vi "Programming Mode.vi"(8 "error in (no error)":errorcluster, 11 "serverName In":string="10.0.18.244") -> (0 "error out":errorcluster, 3 "serverName Out":string="10.0.18.244")   [LabVIEW 2019, in "SEECD System Explorer.lvlib"]
doc: "This VI detects whether or not target local chassis supports \"Slot Programming Mode\" property.\nIf the case, populated slots have current value for the property displayed and user can change property.\nIf not the case, front-panel is not opened."
uses:
  SEECD System Explorer.lvlib
  Type Defs/Slot - Configuration.ctl
  <vilib>/nisyscfg/Close (Resources).vi
  <vilib>/nisyscfg/Close (Filter).vi
  <vilib>/nisyscfg/Close (System).vi
  <vilib>/nisyscfg/nisyscfg.lvlib
panel:
  in  "Slot 7":T1={"Slot"="", "Module Name"="", "Slot Programming Mode"=enum."Don't Modify"} caption="Slot"
  in  "Slot 6":T1={"Slot"="", "Module Name"="", "Slot Programming Mode"=enum."Don't Modify"} caption="Slot"
  in  "Slot 5":T1={"Slot"="", "Module Name"="", "Slot Programming Mode"=enum."Don't Modify"} caption="Slot"
  in  "Slot 4":T1={"Slot"="", "Module Name"="", "Slot Programming Mode"=enum."Don't Modify"} caption="Slot"
  in  "Slot 3":T1={"Slot"="", "Module Name"="", "Slot Programming Mode"=enum."Don't Modify"} caption="Slot"
  in  "Slot 2":T1={"Slot"="", "Module Name"="", "Slot Programming Mode"=enum."Don't Modify"} caption="Slot"
  in  "Slot 1":T1={"Slot"="", "Module Name"="", "Slot Programming Mode"=enum."Don't Modify"} caption="Slot"
  in  "Slot 0":T1={"Slot"="", "Module Name"="", "Slot Programming Mode"=enum."Don't Modify"} caption="Slot"
  in  "User Name":string
  in  "Password":string
  in  "Set all modules to \"Scan Engine\" mode":bool
  in  "Cancel":bool
  in  "OK":bool
  # "Select a programming mode for detected \nmodules and click \"OK\" button."
  # "Module Name"
  # "Programming Mode"
  # "Modules Name"
  # "Slot"
  # "Programming Mode"
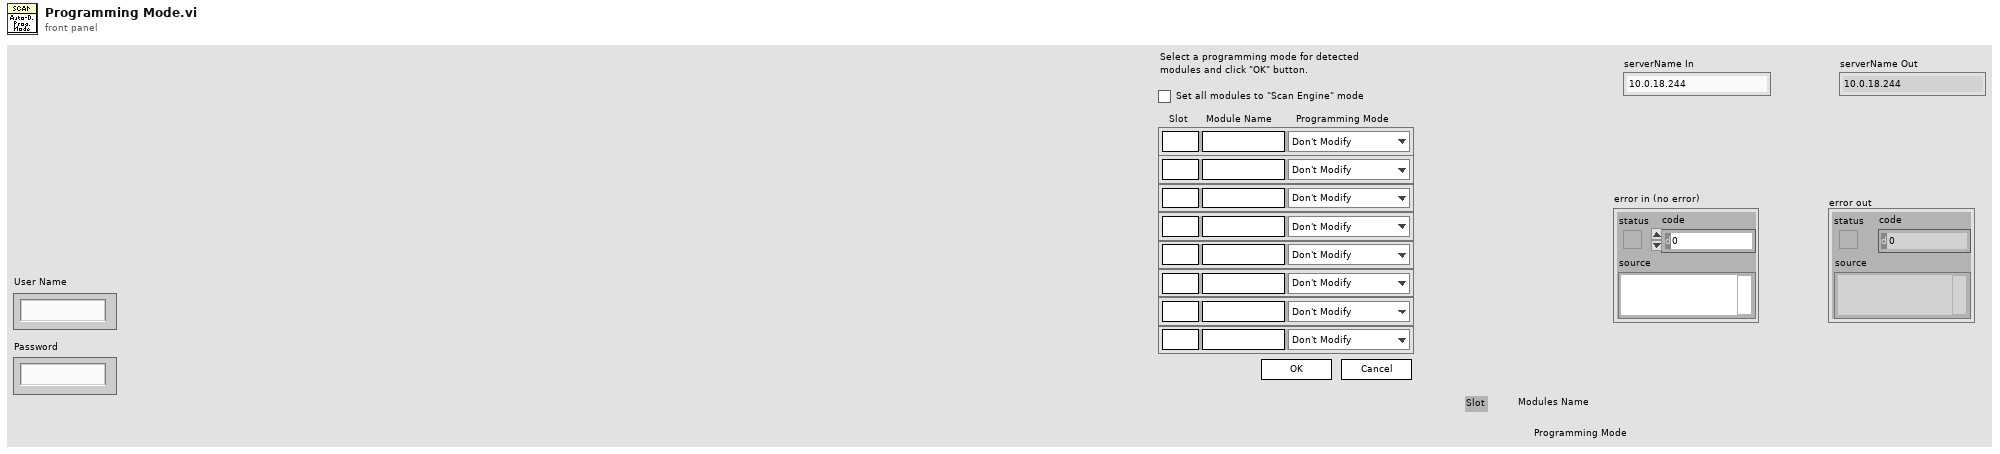
[diagram p1: front panel]
types:
  T1 = typedef "SEECD System Explorer.lvlib/Slot - Configuration.ctl" = cluster{"Slot":string, "Module Name":string, "Slot Programming Mode":enum16{"Scan Engine", "LabVIEW FPGA", "NI-DAQmx", "Don't Modify"}}
  T2 = enum32{"Invalid", "Standard", "Closed", "Hidden", "Minimized", "Maximized"}
  T3 = typedef "SEECD System Explorer.lvlib/Slot Programming Mode.ctl" = enum16{"Scan Engine", "LabVIEW FPGA", "NI-DAQmx", "Don't Modify"}
  T4 = enum16{"Scan Engine", "LabVIEW FPGA", "NI-DAQmx", "Don't Modify"}
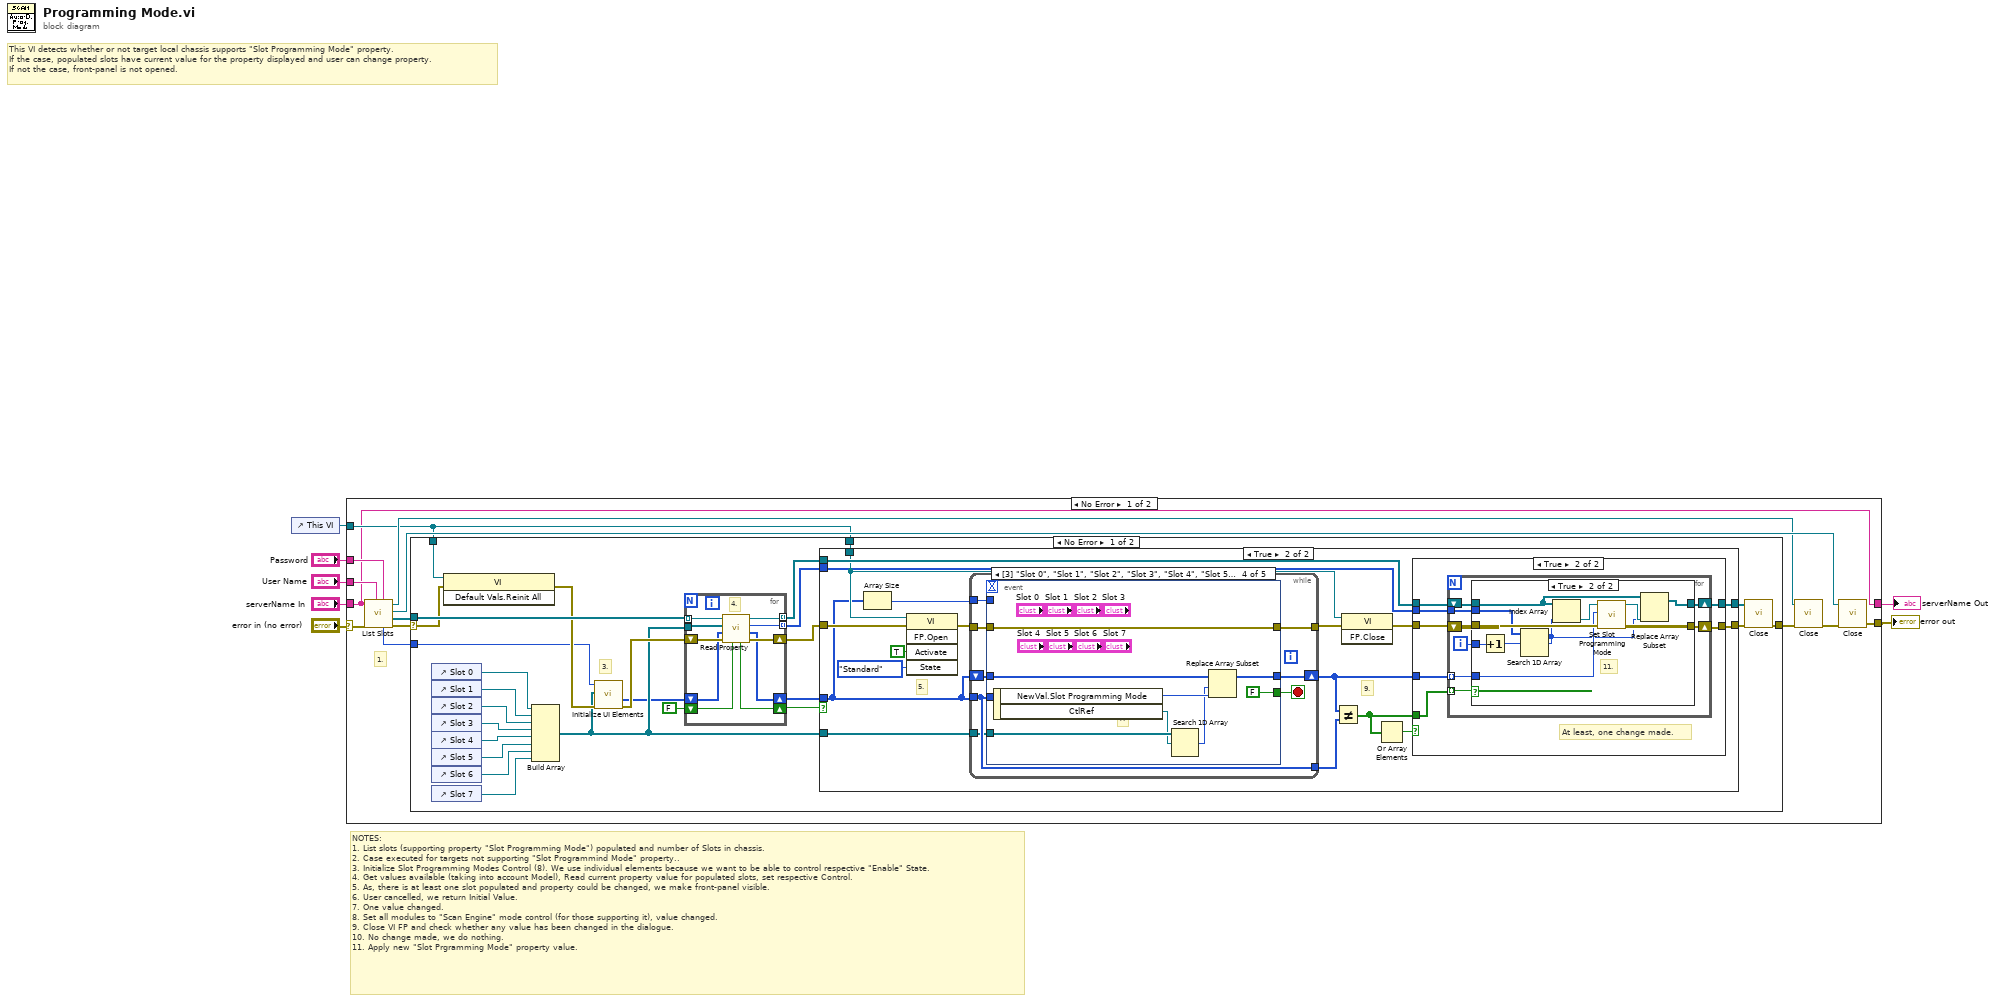
[diagram p0: block diagram]
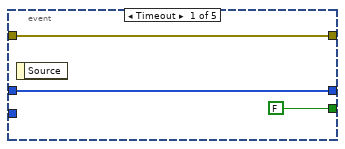
[diagram p3: hidden frame]
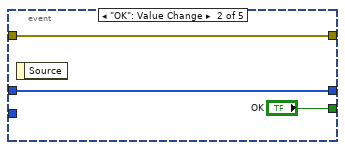
[diagram p4: hidden frame]
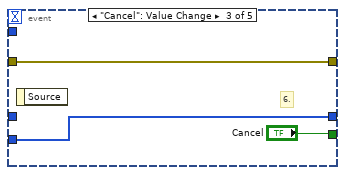
[diagram p5: hidden frame]
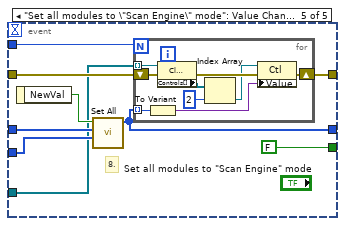
[diagram p6: hidden frame]
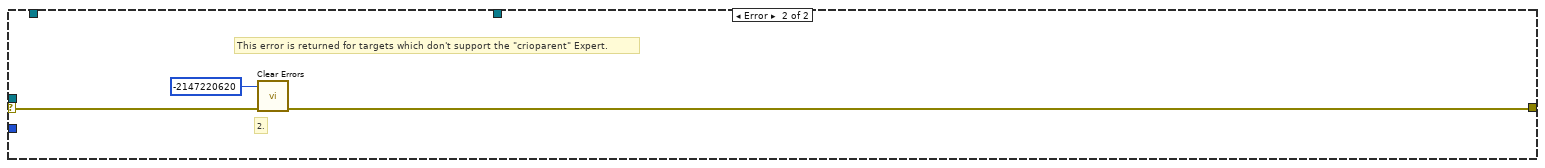
[diagram p9: hidden frame]
diagram:
  # "NOTES:\n1. List slots (supporting property \"Slot Programming Mode\") populated and number of Slots in chassis.\n2. Case executed for targets not supporting \"Slot Programmind Mode\" property..\n3. Initialize Slot Programming Modes Control (8). We use individual elements because we want to be able to control respective \"Enable\" State.\n4. Get values available (taking into account Model), Read current property value for populated slots, set respective Control.\n5. As, there is at least one slot populated and property could be changed, we make front-panel visible.\n6. User cancelled, we return Initial Value.\n7. One value changed.\n8. Set all modules to \"Scan Engine\" mode control (for those supporting it), value changed.\n9. Close VI FP and check whether any value has been changed in the dialogue.\n10. No change made, we do nothing.\n11. Apply new \"Slot Prgramming Mode\" property value."
  # "This VI detects whether or not target local chassis supports \"Slot Programming Mode\" property.\nIf the case, populated slots have current value for the property displayed and user can change property.\nIf not the case, front-panel is not opened."
  n1 = control-ref of="This VI"() -> (w2:refnum<vi>)
  n2 = case shown="No Error" "error in (no error)" {
    selector: "error in (no error)" -> [w19 w154]
    tunnel: "serverName In" -> [w9 w153]
    tunnel: "User Name" -> [w11 _]
    tunnel: "Password" -> [w10 _]
    tunnel: [w20 w154] -> w3
    tunnel: w2 -> [w12 _]
    tunnel: [w9 w153] -> w1
    frame No Error {
      # "1."
      n3 = call "List Slots.vi"("Password"=w10, "User Name"=w11, "error in (no error)"=w19, "serverName In"=w9) -> ("error out"=w14:errorcluster, "Resources out"=w18:refnum<k20>[], "Session out"=w17:refnum<k21>, "Refnum out"=w13:refnum<k20>, "NumSlots"=w8:i32)  [unwired: 3 in]
      n4 = case shown="No Error" w14 {
        selector: w14 -> [w36 w152]
        tunnel: w18 -> [w46 _]
        tunnel: [w42 w150] -> w15
        tunnel: w12 -> [w41 _]
        tunnel: w12 -> [w37 _]
        tunnel: w8 -> [w23 _]
        frame No Error {
          # "3."
          n5 = control-ref of="Slot 0"() -> (w28:refnum<vi>)
          n6 = control-ref of="Slot 1"() -> (w29:refnum<vi>)
          n7 = control-ref of="Slot 2"() -> (w30:refnum<vi>)
          n8 = control-ref of="Slot 3"() -> (w31:refnum<vi>)
          n9 = control-ref of="Slot 4"() -> (w32:refnum<vi>)
          n10 = control-ref of="Slot 5"() -> (w33:refnum<vi>)
          n11 = control-ref of="Slot 6"() -> (w34:refnum<vi>)
          n12 = control-ref of="Slot 7"() -> (w35:refnum<vi>)
          n13 = invoke class="VI" method="Default Vals.Reinit All"(reference=w37, error in=w36) -> (error out=w27:errorcluster)  [unwired: 1 in, 2 out]
          n14 = Build Array(w28, w29, w30, w31, w32, w33, w34, w35) -> (w22:refnum<vi>[])
          n15 = call "Initialize UI Elements.vi"("error in"=w27, "References"=w22, "NumSlots"=w23) -> ("error out"=w26:errorcluster, "Programming Mode Out"=w21:T3[])  [unwired: 7 in]
          n16 = for {
            tunnel: w46 -> [w145] mode=indexing
            shift-right: [w149] -> w43
            shift-left: w26 -> [w148]
            tunnel: [w144] -> w40 mode=indexing
            shift-right: [w141] -> w44
            shift-left: FALSE -> [w147]
            tunnel: w22 -> [w140]
            shift-right: [w142] -> w25
            shift-left: w21 -> [w146]
            tunnel: [w143] -> w24 mode=indexing
            # "4."
            n17 = call "Read Property.vi"("Initialized in"=w147, "error in (no error)"=w148, "Programming Mode In"=w146, "References"=w140, "Refnum in"=w145) -> ("error out"=w149:errorcluster, "Programming Mode Out"=w142:T3[], "Slot"=w143:i32, "Refnum out"=w144:refnum<k20>, "Initialized Out"=w141:bool)  [unwired: 2 in]
          }
          n18 = case shown="True" w44 {
            tunnel: w43 -> [w48 w53]
            tunnel: [w48 w56] -> w38
            tunnel: w25 -> [_ w51]
            tunnel: w41 -> [_ w54]
            tunnel: w40 -> [w47 w61]
            tunnel: [w47 w55] -> w39
            tunnel: w22 -> [_ w52]
            tunnel: w24 -> [_ w49]
            frame False {
            }
            frame True {
              # "9."
              # "5."
              n19 = Array Size(array=w51) -> (size(s)=w50:i32)
              n20 = invoke class="VI" method="FP.Open"(reference=w54, error in=w53, "Activate"=TRUE ("Activate?"), "State"=T2."Standard") -> (error out=w63:errorcluster)  [unwired: 1 in, 4 out]
              n21 = while {
                tunnel: w63 -> [w74]
                tunnel: w51 -> [w71]
                tunnel: [w71] -> w66
                tunnel: [w70] -> w62
                shift-right: [w72] -> w57
                shift-left: w51 -> [w69]
                tunnel: w52 -> [w68]
                tunnel: w50 -> [w67]
                stop <- w73 stop-if-true
                n22 = event shown="[3] \"Slot 0\", \"Slot 1\", \"Slot 2\", \"Slot 3\", \"Slot 4\", \"Slot 5\", \"Slot 6\", \"Slot 7\": Value Change" {
                  selector: _ -> [_ _ _ _ _]
                  dyn-events: _ -> [_ _ _ _ _]
                  timeout: _ -> [_ _ _ _ _]
                  tunnel: w74 -> [w77 w79 w81 w90 w96]
                  tunnel: [FALSE ("Cancel") "OK" "Cancel" FALSE ("Cancel") FALSE ("Cancel")] -> w73
                  tunnel: [w76 w78 w82 w87 w94] -> w72
                  tunnel: w71 -> [_ _ w82 _ w95]
                  tunnel: [w77 w79 w81 w90 w97] -> w70
                  tunnel: w69 -> [w76 w78 _ w89 w98]
                  tunnel: w68 -> [_ _ _ w86 w93]
                  tunnel: w67 -> [_ _ _ _ w92]
                  event Timeout {
                    n23 = event-data() -> ()  [unwired: 1 in, 1 out]
                  }
                  event "OK": Value Change {
                    n24 = event-data() -> ()  [unwired: 1 in, 1 out]
                  }
                  event "Cancel": Value Change {
                    # "6."
                    n25 = event-data() -> ()  [unwired: 1 in, 1 out]
                  }
                  event Value Change {
                    # "7."
                    n26 = event-data() -> ("NewVal.Slot Programming Mode"=w88:T4, "CtlRef"=w84:refnum<vi>)  [unwired: 1 in]
                    n27 = Search 1D Array(1D array=w86, element=w84) -> (index of element=w85:i32)  [unwired: 1 in]
                    n28 = Replace Array Subset(array=w89, new element=w88, index=w85) -> (w87:T3[])
                  }
                  event "Set all modules to \"Scan Engine\" mode": Value Change {
                    # "8."
                    n29 = event-data() -> ("NewVal"=w99:bool)  [unwired: 1 in]
                    n30 = call "Set All.vi"("Init Value"=w95, "Previous Value"=w98, "Set ALL NewVal"=w99) -> ("Value Out"=w94:T3[])  [unwired: 8 in]
                    n31 = for {
                      N: w92 -> [_]
                      tunnel: w94 -> [w102] mode=indexing
                      shift-right: [w103] -> w97
                      shift-left: w96 -> [w109]
                      tunnel: w93 -> [w108] mode=indexing
                      n32 = To Variant(anything=w102) -> (Variant=w101:variant)
                      n33 = property class="Clust (strict)"(reference=w108, error in=w109) -> (error out=w105:errorcluster, "Controls[]"=w107:refnum<vi>[])  [unwired: 1 out]
                      n34 = Index Array(array=w107, index=2) -> (element=w104:refnum<vi>)
                      n35 = property class="Ctl"(reference=w104, error in=w105, "Value"=w101) -> (error out=w103:errorcluster)  [unwired: 1 out]
                    }
                  }
                }
              }
              n36 = Not Equal?(x=w57, y=w66) -> (x != y?=w58:bool[])
              n37 = invoke class="VI" method="FP.Close"(reference=w54, error in=w62) -> (error out=w60:errorcluster)  [unwired: 1 in, 2 out]
              n38 = Or Array Elements(Boolean array=w58) -> (logical OR=w59:bool)
              n39 = case shown="True" w59 {
                tunnel: w61 -> [w110 w118]
                tunnel: w60 -> [w111 w117]
                tunnel: w58 -> [_ w116]
                tunnel: w57 -> [_ w115]
                tunnel: [w111 w114] -> w56
                tunnel: [w110 w113] -> w55
                tunnel: w49 -> [_ w112]
                frame False {
                  # "10."
                  # "Not a single change."
                }
                frame True {
                  # "At least, one change made."
                  n40 = for {
                    tunnel: w116 -> [w126] mode=indexing
                    tunnel: w115 -> [w125] mode=indexing
                    shift-right: [w122] -> w114
                    shift-left: w117 -> [w124]
                    tunnel: w112 -> [w119]
                    shift-right: [w121] -> w113
                    shift-left: w118 -> [w123]
                    i -> [w120]
                    n41 = case shown="True" w126 {
                      tunnel: w125 -> [_ w137]
                      tunnel: w124 -> [w128 w139]
                      tunnel: w123 -> [w127 w131]
                      tunnel: [w128 w138] -> w122
                      tunnel: [w127 w129] -> w121
                      tunnel: w120 -> [_ w135]
                      tunnel: w119 -> [_ w136]
                      frame False {
                      }
                      frame True {
                        # "11."
                        n42 = Increment(x=w135) -> (x+1=w134:i32)
                        n43 = Search 1D Array(1D array=w136, element=w134) -> (index of element=w130:i32)  [unwired: 1 in]
                        n44 = Index Array(array=w131, index=w130) -> (element=w133:refnum<k20>)
                        n45 = call "Set Slot Programming Mode.vi"("error in (no error)"=w139, "Slot Programming Mode"=w137, "Refnum in"=w133) -> ("error out"=w138:errorcluster, "Refnum out"=w132:refnum<k20>)  [unwired: 7 in]
                        n46 = Replace Array Subset(array=w131, new element=w132, index=w130) -> (w129:refnum<k20>[])
                      }
                    }
                  }
                }
              }
            }
          }
          n47 = call-poly <vilib>:"Close.vi"("error in (no error)"=w38, "Resources in"=w39) -> ("error out"=w42:errorcluster)  [unwired: 9 in]
        }
        frame Error {
          # "2."
          # "This error is returned for targets which don't support the \"crioparent\" Expert."
          n48 = call <vilib>:"Clear Errors.vi"("error in (no error)"=w152, "specific error code to clear (0: all)"=-2147220620) -> ("error out"=w150:errorcluster)  [unwired: 4 in, 1 out]
        }
      }
      n49 = call-poly <vilib>:"Close.vi"("error in (no error)"=w15, "Filter in"=w13) -> ("error out"=w16:errorcluster)  [unwired: 9 in]
      n50 = call-poly <vilib>:"Close.vi"("error in (no error)"=w16, "Session in"=w17) -> ("error out"=w20:errorcluster)  [unwired: 9 in]
    }
    frame Error {
    }
  }
  "error out" <- w3
  "serverName Out" <- w1
